vi "GOOP_DesignPatternPathFix.vi"(11 "ViPathIn":path) -> (0 "RelativeVIPathOut(ToStoreInLvClass)":path, 1 "Ini-File":path, 2 "Folder":path, 3 "ViPathOut":path, 5 "Found":bool)   [LabVIEW 2016]
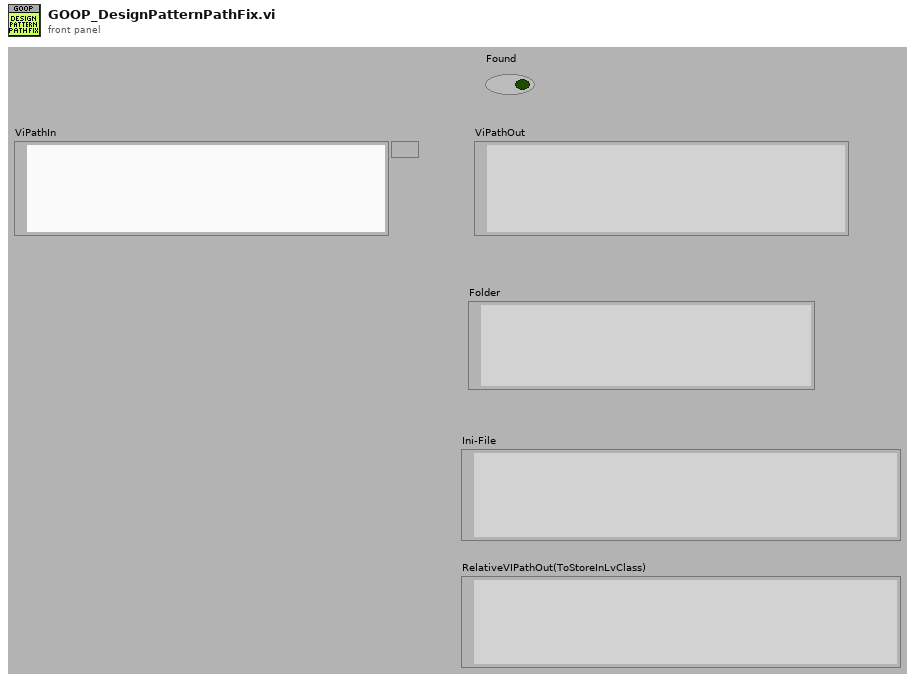
[diagram p1: front panel]
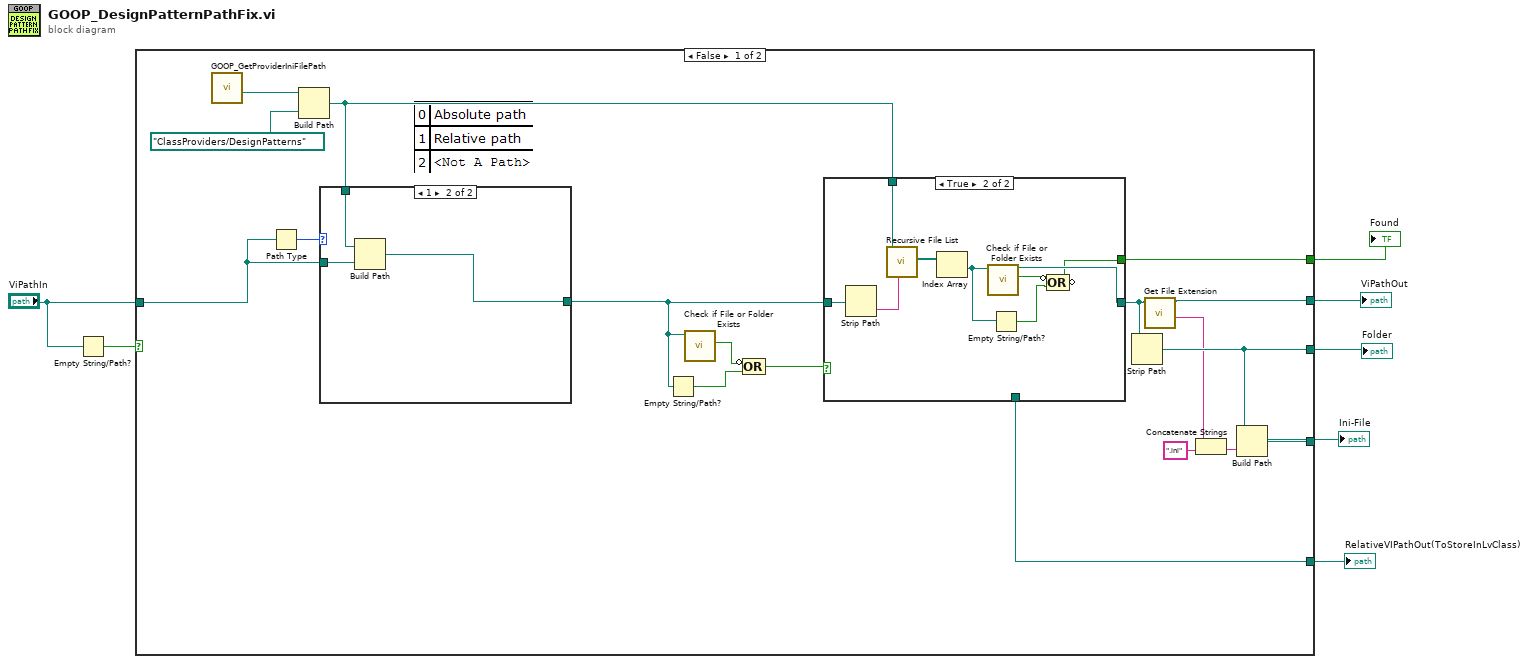
[diagram p0: block diagram]
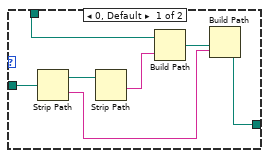
[diagram p2: hidden frame]
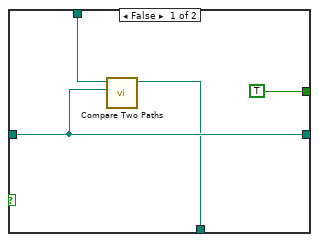
[diagram p3: hidden frame]
diagram:
  n1 = Empty String/Path?(string/path="ViPathIn") -> (empty?=w1:bool)
  n2 = case shown="False" w1 {
    tunnel: [w25 _] -> w7
    tunnel: [w24 _] -> w6
    tunnel: [w19 _] -> w5
    tunnel: [w18 _] -> w4
    tunnel: [w13 _] -> w3
    tunnel: "ViPathIn" -> [w8 _]
    frame False {
      n3 = call <resource>:"GOOP_GetProviderIniFilePath.vi"() -> ("ProviderMainFolder"=w17:path)  [unwired: 10 in, 1 out]
      n4 = Path Type(1:w8) -> (0:w15:i16)
      n5 = Build Path(base path=w17, name or relative path=path "ClassProviders/DesignPatterns" ("base path")) -> (appended path=w14:path)
      n6 = case shown="1" w15 {
        tunnel: w14 -> [w30 w35]
        tunnel: w8 -> [w32 w34]
        tunnel: [w26 w33] -> w12
        frame 0, Default {
          n7 = Strip Path(path=w32) -> (stripped path=w31:path, name=w27:string)
          n8 = Strip Path(path=w31) -> (name=w29:string)  [unwired: 1 out]
          n9 = Build Path(base path=w30, name or relative path=w29) -> (appended path=w28:path)
          n10 = Build Path(base path=w28, name or relative path=w27) -> (appended path=w26:path)
        }
        frame 1 {
          n11 = Build Path(base path=w35, name or relative path=w34) -> (appended path=w33:path)
        }
      }
      n12 = Empty String/Path?(string/path=w12) -> (empty?=w10:bool)
      n13 = call <vilib>:"Check if File or Folder Exists.vi"("path"=w12) -> ("file or folder exists?"=w11:bool)  [unwired: 8 in, 2 out]
      n14 = Compound Arithmetic op=OR(invert w11, w10) -> (w9:bool)
      n15 = case shown="True" w9 {
        tunnel: w12 -> [w37 w47]
        tunnel: [w37 w44] -> w20
        tunnel: [TRUE w40] -> w19
        tunnel: w14 -> [w38 w48]
        tunnel: [w36 _] -> w13
        frame False {
          n16 = call <vilib>:"Compare Two Paths.vi"("Path 2"=w37, "Path 1"=w38) -> ("Relative Path from 1 to 2"=w36:path)  [unwired: 6 in, 3 out]
        }
        frame True {
          n17 = Strip Path(path=w47) -> (name=w46:string)  [unwired: 1 out]
          n18 = call <vilib>:"Recursive File List.vi"("pattern"=w46, "Folder Path"=w48) -> ("All Files in Dir"=w45:path[])  [unwired: 5 in, 4 out]
          n19 = Index Array(array=w45) -> (element=w42:path)  [unwired: 1 in]
          n20 = call <vilib>:"Check if File or Folder Exists.vi"("path"=w42) -> ("file or folder exists?"=w43:bool, "dup path"=w44:path)  [unwired: 8 in, 1 out]
          n21 = Empty String/Path?(string/path=w42) -> (empty?=w41:bool)
          n22 = Compound Arithmetic op=OR(invert w43, w41) -> (invert w40:bool)
        }
      }
      n23 = Strip Path(path=w20) -> (stripped path=w24:path)  [unwired: 1 out]
      n24 = call <vilib>:"Get File Extension.vi"("file"=w20) -> ("filename without extension"=w21:string, "dup file"=w18:path)  [unwired: 6 in, 3 out]
      n25 = Concatenate Strings(w21, ".ini" ("string")) -> (w23:string)
      n26 = Build Path(base path=w24, name or relative path=w23) -> (appended path=w25:path)
    }
    frame True {
    }
  }
  "Ini-File" <- w7
  "Folder" <- w6
  "ViPathOut" <- w4
  "Found" <- w5
  "RelativeVIPathOut(ToStoreInLvClass)" <- w3
